vi "FL_Calculate_Coordinates_for_saving.vi"(3 "Magnets coords in":T1) -> (1 "Output cluster of data":T2)   [LabVIEW 2016]
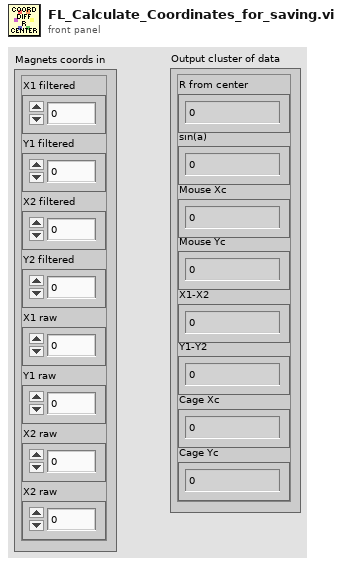
[diagram p1: front panel]
types:
  T1 = cluster{"X1 filtered":dbl, "Y1 filtered":dbl, "X2 filtered":dbl, "Y2 filtered":dbl, "X1 raw":dbl, "Y1 raw":dbl, "X2 raw":dbl, "X2 raw":dbl}
  T2 = cluster{"R from center":dbl, "sin(a)":dbl, "Mouse Xc":dbl, "Mouse Yc":dbl, "X1-X2":dbl, "Y1-Y2":dbl, "Cage Xc":dbl, "Cage Yc":dbl}
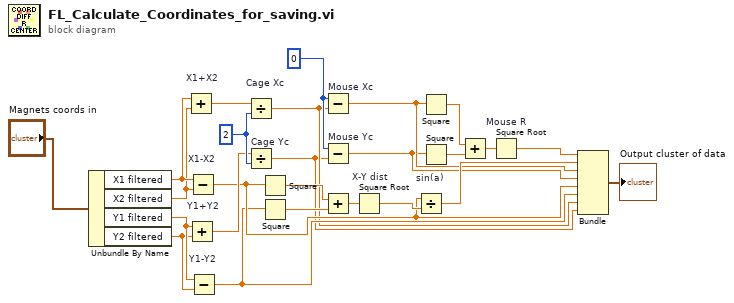
[diagram p0: block diagram]
diagram:
  w15 = 0
  w18 = 2
  n1 = Unbundle By Name("Magnets coords in") -> ("X1 filtered"=w14:dbl, "X2 filtered"=w13:dbl, "Y1 filtered"=w12:dbl, "Y2 filtered"=w11:dbl)
  n2 = Add "X1+X2"(x=w14, y=w13) -> (x+y=w16:dbl)
  n3 = Add "Y1+Y2"(x=w12, y=w11) -> (x+y=w17:dbl)
  n4 = Subtract "X1-X2"(x=w14, y=w13) -> (x-y=w6:dbl)
  n5 = Subtract "Y1-Y2"(x=w12, y=w11) -> (x-y=w5:dbl)
  n6 = Divide "Cage Xc"(x=w16, y=w18) -> (x/y=w4:dbl)
  n7 = Divide "Cage Yc"(x=w17, y=w18) -> (x/y=w3:dbl)
  n8 = Square(x=w6) -> (x^2=w19:dbl)
  n9 = Square(x=w5) -> (x^2=w20:dbl)
  n10 = Subtract "Mouse Xc"(x=w15, y=w4) -> (x-y=w8:dbl)
  n11 = Subtract "Mouse Yc"(x=w15, y=w3) -> (x-y=w7:dbl)
  n12 = Add(x=w19, y=w20) -> (x+y=w21:dbl)
  n13 = Square Root "X-Y dist"(x=w21) -> (sqrt(x)=w22:dbl)
  n14 = Divide "sin(a)"(x=w6, y=w22) -> (x/y=w9:dbl)
  n15 = Square(x=w8) -> (x^2=w23:dbl)
  n16 = Square(x=w7) -> (x^2=w24:dbl)
  n17 = Add(x=w23, y=w24) -> (x+y=w25:dbl)
  n18 = Square Root "Mouse R"(x=w25) -> (sqrt(x)=w10:dbl)
  n19 = Bundle(w10, w9, w8, w7, w6, w5, w4, w3) -> (→"Output cluster of data":cluster{dbl, dbl, dbl, dbl, dbl, dbl, dbl, dbl})  [unwired: 1 in]
